vi "OBE_ODMR_demo.vi"() -> ()   [LabVIEW 2015]
uses:
  states.ctl
panel:
  in  "Where's OBETCP.py?":path=path "C:/Users/rdm/Desktop/obe-one/optimized-bayes-experimental-design/Demos/LabView/lorentz_OBETCP.py"
  out "B array":dbl[](array[numeric])
  out "sim params":T1
  in  "Nvals B":i32=51
  in  "Stop B":dbl=225000.0
  in  "Start B":dbl=175000.0
  in  "background":dbl=200000.0
  out "A array":dbl[](array[numeric])
  in  "Nvals A":i32=101
  in  "Stop A":dbl=-40000.0
  in  "Start A":dbl=-5000.0
  in  "Amplitude":dbl
  out "size(s)":i32
  out "sim. y":dbl
  out "X copy":dbl
  out "true curve":cluster{"X Array":dbl[], dbl[]}
  in  "stopmeas":bool
  in  "stop":bool
  out "X Array":dbl[](array[numeric])
  out "X0 Array":dbl[](array[numeric])
  in  "Nvals X0":i32=101
  in  "Stop X0":dbl=4.0
  in  "Start X0":dbl=2.0
  in  "Nvals X":i32=51
  in  "Stop X":dbl=4.5
  in  "Start X":dbl=1.5
  in  "run":bool
  out "error out":errorcluster
  in  "error in (no error)":errorcluster
  out "plots":cluster{"X Array":dbl[], "ydata":dbl[]}[](graph)
  in  "randomize":bool
  in  "setup":bool
  in  "Resonance frequency":dbl
  in  "Width":dbl=0.1
  # "Measurement settings"
  # "Resonance freq parameter"
  # "Peak Amplitude"
  # "Background"
  # "Constants"
  # "Secret \"true\" values"
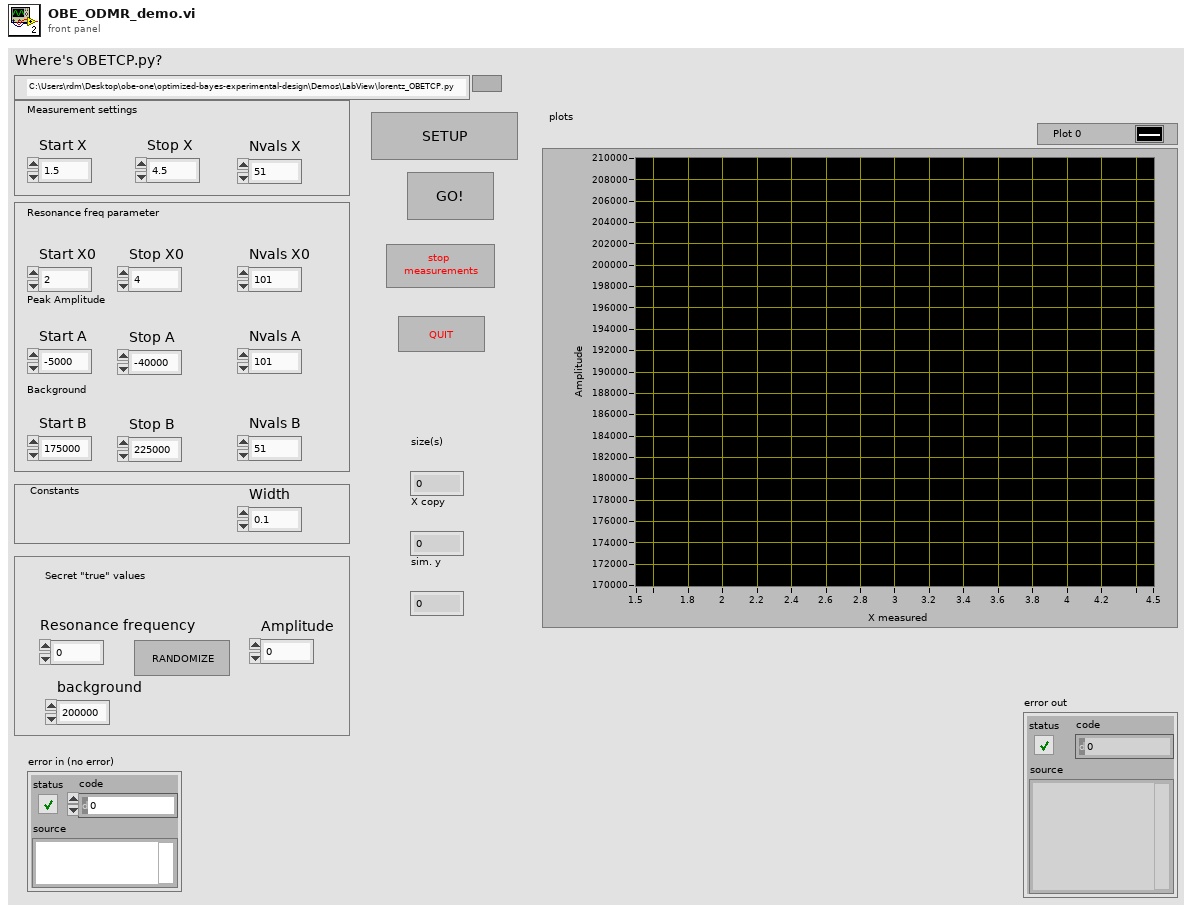
[diagram p1: front panel]
types:
  T1 = cluster{"Resonance frequency":dbl, "Amplitude":dbl, "background":dbl, "Width":dbl}
  T2 = typedef "states.ctl" = enum16{"Idle", "initialize", "randomize", "setup", "run", "wrapup", "shutdown"}
  T3 = enum16{"clrset", "clrpar", "clrcon", "getset", "getpar", "getcon", "addset", "addpar", "addcon", "config", "done"}
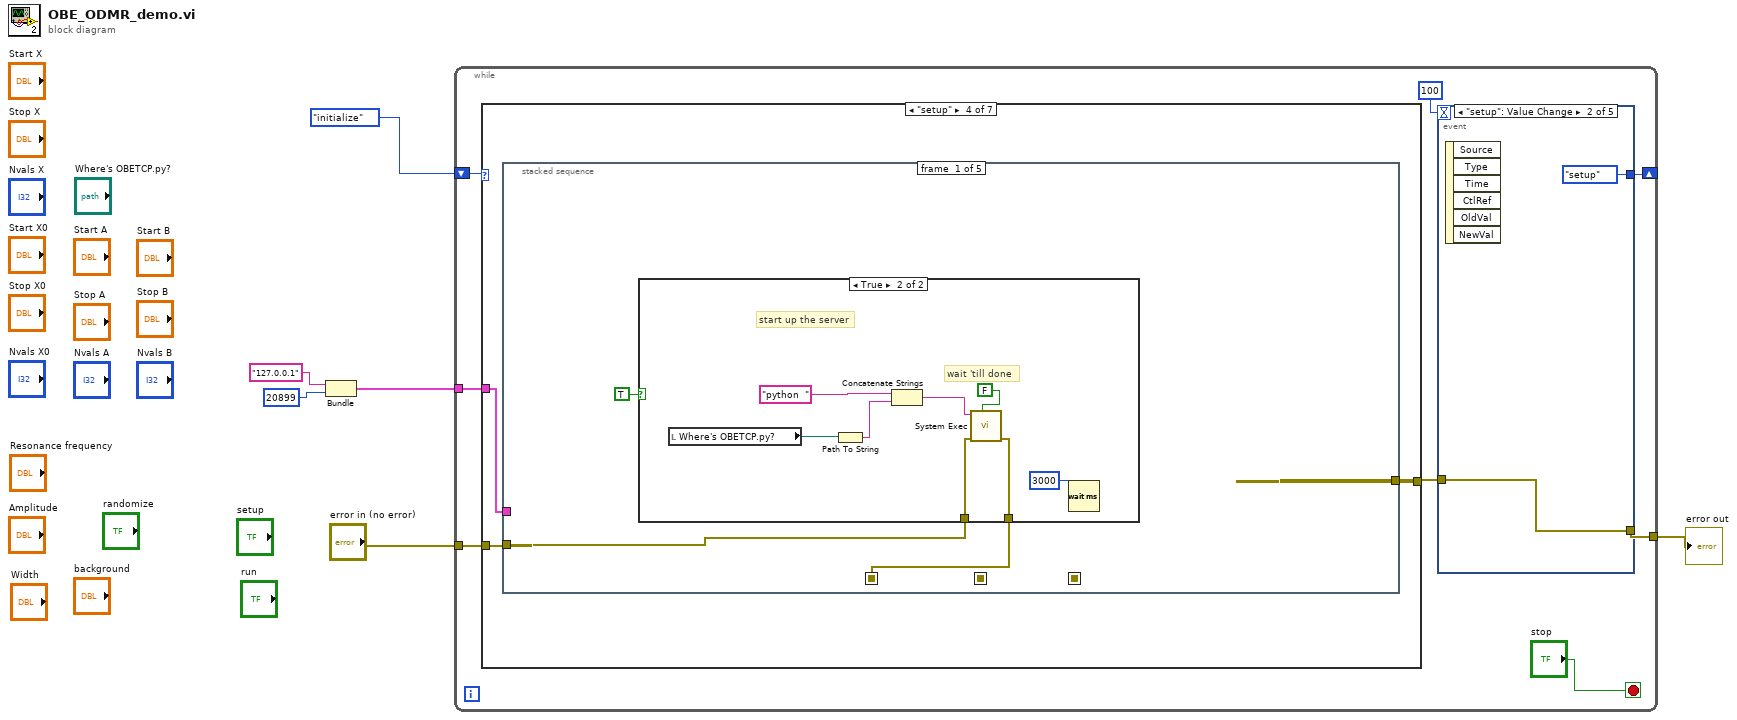
[diagram p0: block diagram]
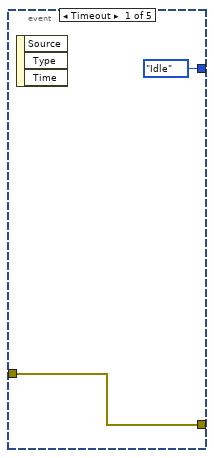
[diagram p2: hidden frame]
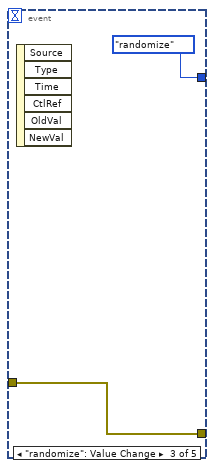
[diagram p3: hidden frame]
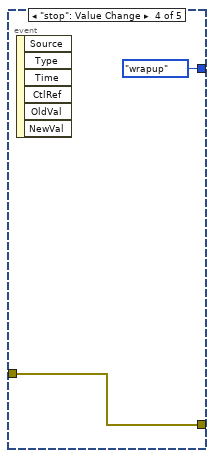
[diagram p4: hidden frame]
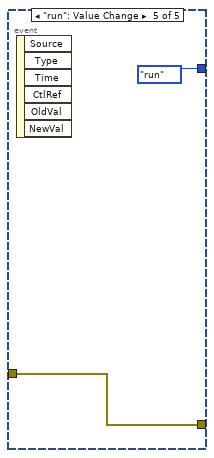
[diagram p5: hidden frame]
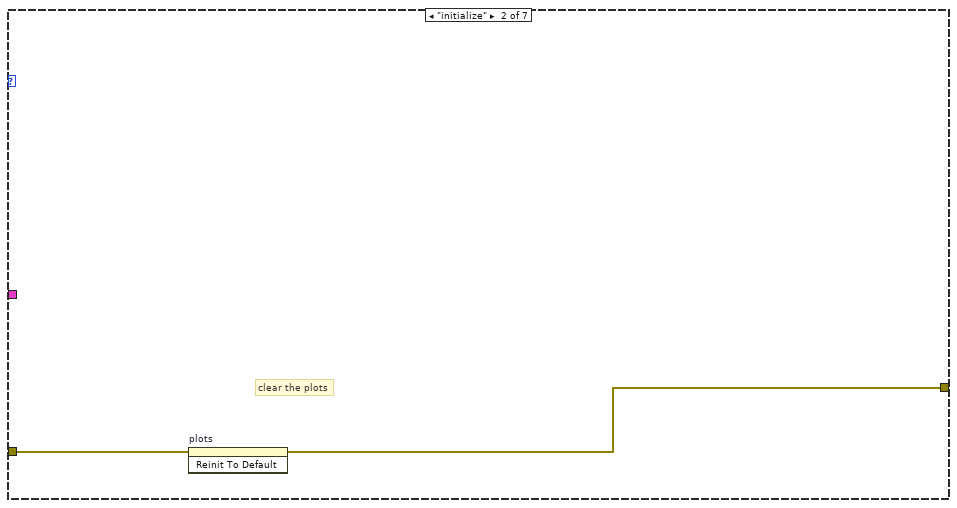
[diagram p7: hidden frame]
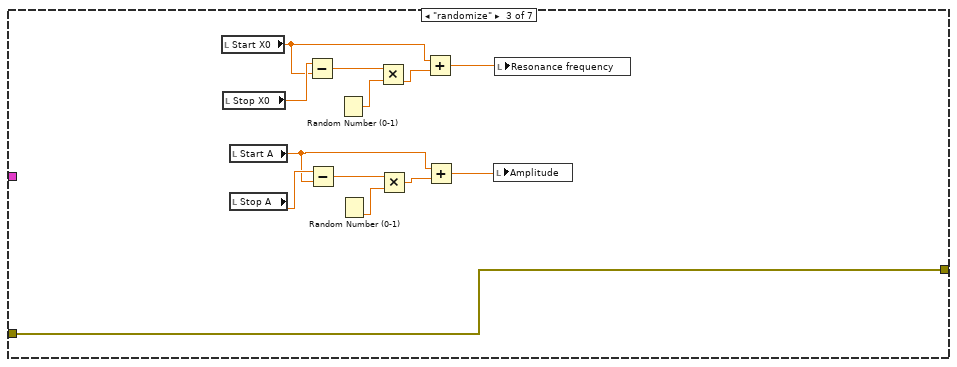
[diagram p8: hidden frame]
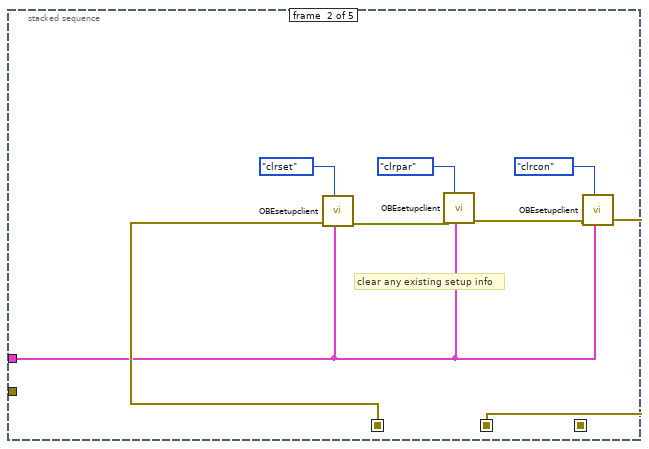
[diagram p10: hidden frame]
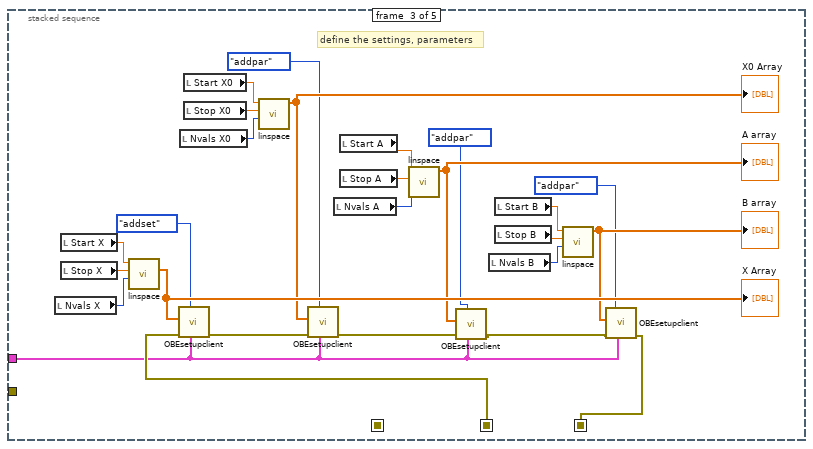
[diagram p11: hidden frame]
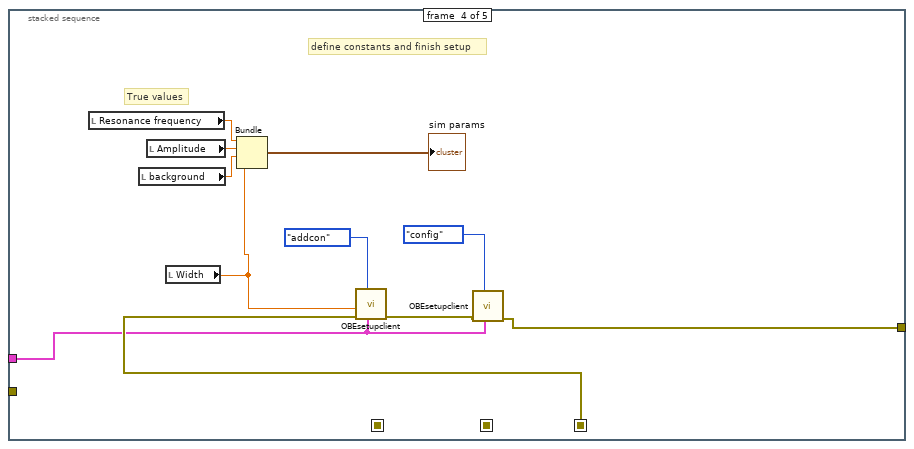
[diagram p12: hidden frame]
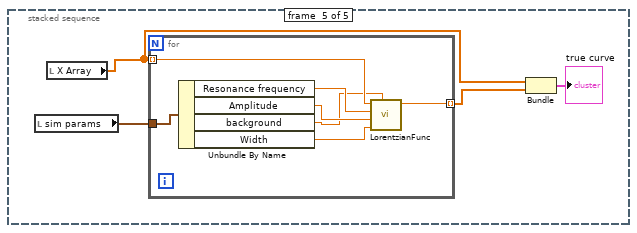
[diagram p13: hidden frame]
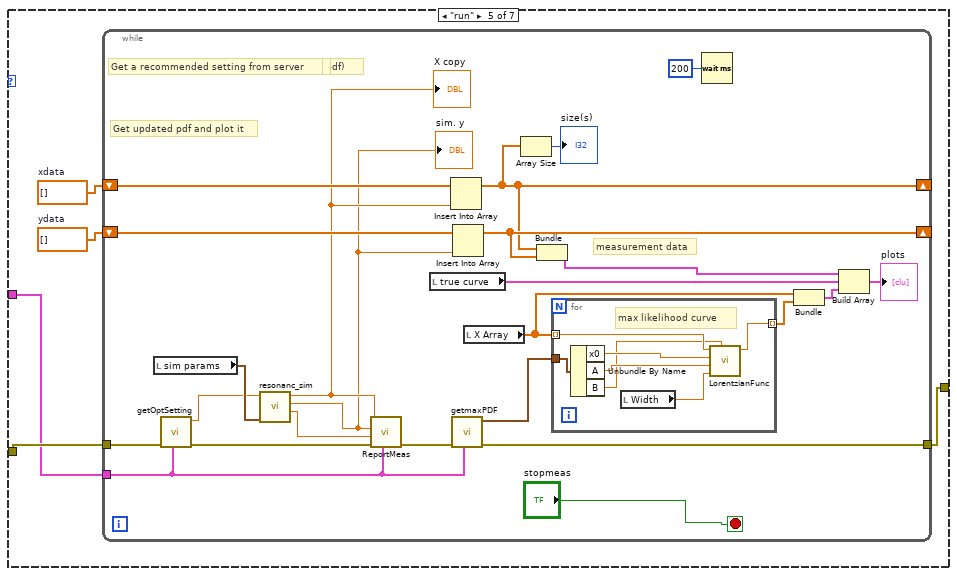
[diagram p14: hidden frame]
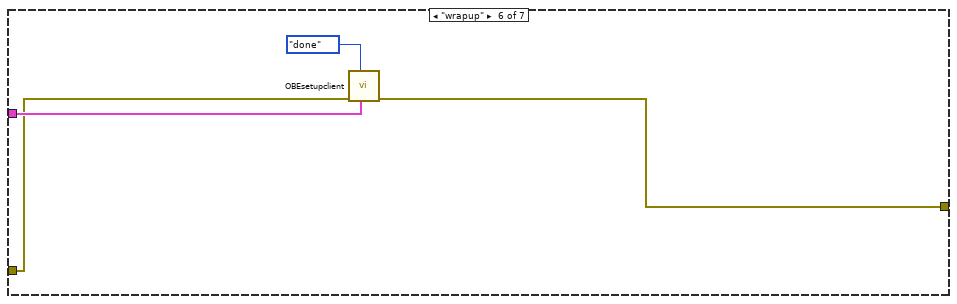
[diagram p15: hidden frame]
diagram:
  n1 = Bundle("127.0.0.1", 20899) -> (w1:cluster{string, i32})  [unwired: 1 in]
  n2 = while {
    shift-right: [w13] -> _
    shift-left: states."initialize" ("states") -> [w14]
    tunnel: "error in (no error)" -> [w12]
    tunnel: [w11] -> w4
    tunnel: w1 -> [w7]
    stop <- "stop" stop-if-true
    n3 = case shown="\"setup\"" w14 {
      tunnel: w12 -> [w25 w27 w36 w43 w116 w150 w152]
      tunnel: [w25 w26 w36 w42 w112 w149 w152] -> w10
      tunnel: w7 -> [_ _ _ w41 w113 w151 _]
      frame "Idle", Default {
      }
      frame "initialize" {
        # "clear the plots"
        n4 = invoke on="plots" class="XYGraph (strict)" method="Reinit To Default"(error in=w27) -> (error out=w26:errorcluster)  [unwired: 2 in, 2 out]
      }
      frame "randomize" {
        n5 = local read "Start X0"() -> (w34:dbl)
        n6 = local read "Stop X0"() -> (w35:dbl)
        n7 = local read "Start A"() -> (w29:dbl)
        n8 = local read "Stop A"() -> (w30:dbl)
        n9 = Subtract(x=w35, y=w34) -> (x-y=w39:dbl)
        n10 = Subtract(x=w30, y=w29) -> (x-y=w32:dbl)
        n11 = Random Number (0-1)() -> (number: 0 to 1=w40:dbl)
        n12 = Random Number (0-1)() -> (number: 0 to 1=w33:dbl)
        n13 = Multiply(x=w39, y=w40) -> (x*y=w38:dbl)
        n14 = Multiply(x=w32, y=w33) -> (x*y=w31:dbl)
        n15 = Add(x=w34, y=w38) -> (x+y=w37:dbl)
        n16 = Add(x=w29, y=w31) -> (x+y=w28:dbl)
        n17 = local write "Amplitude"(w28) -> ()
        n18 = local write "Resonance frequency"(w37) -> ()
      }
      frame "setup" {
        n19 = stacked-sequence {
          seq-local: [w45 _ _ _ _] -> [_ w63 _ _ _]
          seq-local: [_ w61 _ _ _] -> [_ _ w82 _ _]
          seq-local: [_ _ w68 _ _] -> [_ _ _ w96 _]
          tunnel: [_ _ _ w92 _] -> w42
          tunnel: w43 -> [w46 _ _ _ _]
          tunnel: w41 -> [_ w56 w67 w90 _]
          frame #0 {
            n20 = case shown="True" TRUE {
              tunnel: w46 -> [w47 w53]
              tunnel: [w47 w52] -> w45
              frame False {
              }
              frame True {
                # "wait 'till done"
                # "start up the server"
                n21 = local read "Where's OBETCP.py?"() -> (w49:path)
                n22 = Path To String(path=w49) -> (string=w48:string)
                n23 = Concatenate Strings("python  " ("command line"), w48) -> (w50:string)
                n24 = call <vilib>:"System Exec.vi"("wait until completion? (T)"=FALSE, "error in (no error)"=w53, "command line"=w50) -> ("error out"=w52:errorcluster)  [unwired: 5 in, 3 out]
                n25 = Wait (ms)(milliseconds to wait=u32 3000) -> ()  [unwired: 1 out]
              }
            }
          }
          frame #1 {
            # "clear any existing setup info"
            n26 = call "OBEsetupclient.vi"("addr/port"=w56, "OBE commands"=T3."clrset" ("BOE commands"), "error in (no error)"=w63) -> ("error out"=w62:errorcluster)  [unwired: 7 in, 1 out]
            n27 = call "OBEsetupclient.vi"("addr/port"=w56, "OBE commands"=T3."clrpar" ("BOE commands"), "error in (no error)"=w62) -> ("error out"=w59:errorcluster)  [unwired: 7 in, 1 out]
            n28 = call "OBEsetupclient.vi"("addr/port"=w56, "OBE commands"=T3."clrcon" ("BOE commands"), "error in (no error)"=w59) -> ("error out"=w61:errorcluster)  [unwired: 7 in, 1 out]
          }
          frame #2 {
            # "define the settings, parameters"
            n29 = local read "Nvals X"() -> (w86:i32)
            n30 = local read "Start X"() -> (w88:dbl)
            n31 = local read "Stop X"() -> (w87:dbl)
            n32 = call "linspace.vi"("Nvalues"=w86, "Stop"=w87, "Start"=w88) -> ("Array"=w89:dbl[])  [unwired: 8 in]
            "X Array" <- w89
            n33 = call "OBEsetupclient.vi"("addr/port"=w67, "OBE commands"=T3."addset" ("BOE commands"), "error in (no error)"=w82, "array"=w89) -> ("error out"=w74:errorcluster)  [unwired: 6 in, 1 out]
            n34 = local read "Nvals X0"() -> (w83:i32)
            n35 = local read "Start X0"() -> (w85:dbl)
            n36 = local read "Stop X0"() -> (w84:dbl)
            n37 = call "linspace.vi"("Nvalues"=w83, "Stop"=w84, "Start"=w85) -> ("Array"=w73:dbl[])  [unwired: 8 in]
            "X0 Array" <- w73
            n38 = call "OBEsetupclient.vi"("addr/port"=w67, "OBE commands"=T3."addpar" ("BOE commands"), "error in (no error)"=w74, "array"=w73) -> ("error out"=w69:errorcluster)  [unwired: 6 in, 1 out]
            n39 = local read "Nvals A"() -> (w78:i32)
            n40 = local read "Start A"() -> (w80:dbl)
            n41 = local read "Stop A"() -> (w79:dbl)
            n42 = call "linspace.vi"("Nvalues"=w78, "Stop"=w79, "Start"=w80) -> ("Array"=w71:dbl[])  [unwired: 8 in]
            "A array" <- w71
            n43 = call "OBEsetupclient.vi"("addr/port"=w67, "OBE commands"=T3."addpar" ("BOE commands"), "error in (no error)"=w69, "array"=w71) -> ("error out"=w64:errorcluster)  [unwired: 6 in, 1 out]
            n44 = local read "Nvals B"() -> (w75:i32)
            n45 = local read "Start B"() -> (w77:dbl)
            n46 = local read "Stop B"() -> (w76:dbl)
            n47 = call "linspace.vi"("Nvalues"=w75, "Stop"=w76, "Start"=w77) -> ("Array"=w66:dbl[])  [unwired: 8 in]
            "B array" <- w66
            n48 = call "OBEsetupclient.vi"("addr/port"=w67, "OBE commands"=T3."addpar" ("BOE commands"), "error in (no error)"=w64, "array"=w66) -> ("error out"=w68:errorcluster)  [unwired: 6 in, 1 out]
          }
          frame #3 {
            # "True values"
            # "define constants and finish setup"
            n49 = local read "Resonance frequency"() -> (w100:dbl)
            n50 = local read "background"() -> (w98:dbl)
            n51 = local read "Amplitude"() -> (w99:dbl)
            n52 = local read "Width"() -> (w95:dbl)
            n53 = Bundle("Resonance frequency"=w100, "Amplitude"=w99, "background"=w98, "Width"=w95) -> (→"sim params":T1)  [unwired: 1 in]
            n54 = call "OBEsetupclient.vi"("addr/port"=w90, "OBE commands"=T3."addcon" ("BOE commands"), "error in (no error)"=w96, "value"=w95) -> ("error out"=w93:errorcluster)  [unwired: 6 in, 1 out]
            n55 = call "OBEsetupclient.vi"("addr/port"=w90, "OBE commands"=T3."config" ("BOE commands"), "error in (no error)"=w93) -> ("error out"=w92:errorcluster)  [unwired: 7 in, 1 out]
          }
          frame #4 {
            n56 = local read "sim params"() -> (w101:T1)
            n57 = local read "X Array"() -> (w103:dbl[])
            n58 = for {
              tunnel: w103 -> [w111] mode=indexing
              tunnel: [w110] -> w104 mode=indexing
              tunnel: w101 -> [w109]
              n59 = Unbundle By Name(w109) -> ("Resonance frequency"=w106:dbl, "Amplitude"=w107:dbl, "background"=w105:dbl, "Width"=w108:dbl)
              n60 = call "LorentzianFunc.vi"("B"=w105, "d"=w108, "A"=w107, "x0"=w106, "X"=w111) -> ("B+A/[1+(X-X0)^2 / d^2]"=w110:dbl)  [unwired: 6 in]
            }
            n61 = Bundle("X Array"=w103, w104) -> (→"true curve":cluster{"X Array":dbl[], dbl[]})  [unwired: 1 in]
          }
        }
      }
      frame "run" {
        w115 = dbl[] []  # ydata
        w114 = dbl[] []  # xdata
        n62 = while {
          tunnel: w116 -> [w137]
          shift-right: [w126] -> _
          shift-left: w114 -> [w136]
          shift-right: [w132] -> _
          shift-left: w115 -> [w135]
          tunnel: w113 -> [w124]
          tunnel: [w122] -> w112
          stop <- "stopmeas" stop-if-true
          # "measurement data"
          # "Get updated pdf and plot it"
          # "Report measurement result (server updates pdf)"
          # "Make (simulate) a measurement  + plot it"
          # "Get a recommended setting from server"
          n63 = local read "sim params"() -> (w139:T1)
          n64 = call "getOptSetting.vi"("addr/port"=w124, "error in (no error)"=w137) -> ("error out"=w140:errorcluster, "setting"=w138:dbl)  [unwired: 8 in]
          n65 = call "resonanc_sim.vi"("sim params"=w139, "X"=w138) -> ("noise estimate"=w117:dbl, "sim. y"=w133:dbl, "X copy"=w134:dbl)  [unwired: 7 in]
          "X copy" <- w134
          "sim. y" <- w133
          n66 = call "ReportMeas.vi"("addr/port"=w124, "error in (no error)"=w140, "s"=w117, "y"=w133, "x"=w134) -> ("error out"=w123:errorcluster)  [unwired: 5 in, 1 out]
          n67 = local read "true curve"() -> (w129:cluster{"X Array":dbl[], dbl[]})
          n68 = Insert Into Array(array=w136, new element=w134) -> (w126:dbl[])  [unwired: 1 in]
          n69 = call "getmaxPDF.vi"("addr/port"=w124, "error in (no error)"=w123) -> ("error out"=w122:errorcluster, "maxparams"=w118:cluster{"x0":dbl, "A":dbl, "B":dbl})  [unwired: 8 in]
          n70 = Insert Into Array(array=w135, new element=w133) -> (w132:dbl[])  [unwired: 1 in]
          n71 = local read "X Array"() -> (w121:dbl[])
          n72 = Array Size(array=w126) -> (size(s)=→"size(s)":i32)
          n73 = Bundle("xdata"=w126, "ydata"=w132) -> (w128:cluster{"xdata":dbl[], "ydata":dbl[]})  [unwired: 1 in]
          n74 = for {
            tunnel: w121 -> [w147] mode=indexing
            tunnel: [w143] -> w120 mode=indexing
            tunnel: w118 -> [w142]
            # "max likelihood curve"
            n75 = Unbundle By Name(w142) -> ("x0"=w146:dbl, "A"=w145:dbl, "B"=w141:dbl)
            n76 = local read "Width"() -> (w144:dbl)
            n77 = call "LorentzianFunc.vi"("B"=w141, "d"=w144, "A"=w145, "x0"=w146, "X"=w147) -> ("B+A/[1+(X-X0)^2 / d^2]"=w143:dbl)  [unwired: 6 in]
          }
          n78 = Wait (ms)(milliseconds to wait=u32 200) -> ()  [unwired: 1 out]
          n79 = Bundle("X Array"=w121, w120) -> (w119:cluster{"X Array":dbl[], dbl[]})  [unwired: 1 in]
          n80 = Build Array(w128, w129, w119) -> (→"plots":cluster{"X Array":dbl[], "ydata":dbl[]}[])
        }
      }
      frame "wrapup" {
        n81 = call "OBEsetupclient.vi"("addr/port"=w151, "OBE commands"=T3."done" ("BOE commands"), "error in (no error)"=w150) -> ("error out"=w149:errorcluster)  [unwired: 7 in, 1 out]
      }
      frame "shutdown" {
      }
    }
    n82 = event shown="[1] \"setup\": Value Change" {
      selector: _ -> [_ _ _ _ _]
      dyn-events: _ -> [_ _ _ _ _]
      timeout: 100 -> [_ _ _ _ _]
      tunnel: [states."Idle" ("states") states."setup" ("states") states."randomize" ("states") states."wrapup" ("states") states."run" ("states")] -> w13
      tunnel: [w16 w17 w19 w21 w23] -> w11
      tunnel: w10 -> [w16 w17 w19 w21 w23]
      event Timeout {
        n83 = event-data() -> ()  [unwired: 1 in, 3 out]
      }
      event "setup": Value Change {
        n84 = event-data() -> ()  [unwired: 1 in, 6 out]
      }
      event "randomize": Value Change {
        n85 = event-data() -> ()  [unwired: 1 in, 6 out]
      }
      event "stop": Value Change {
        n86 = event-data() -> ()  [unwired: 1 in, 6 out]
      }
      event "run": Value Change {
        n87 = event-data() -> ()  [unwired: 1 in, 6 out]
      }
    }
  }
  "error out" <- w4
